vi "is-serial-port-open.vi"(11 "VISA Refnum in":refnum<visa-resource-name>) -> (0 "port-status":bool)   [LabVIEW 2024]
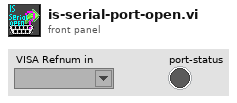
[diagram p1: front panel]
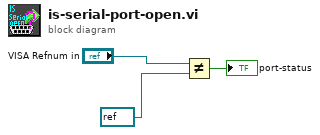
[diagram p0: block diagram]
diagram:
  n1 = Not Equal?(x="VISA Refnum in", y=refnum<visa-resource-name> refnum ("VISA resource name out")) -> (x != y?=→"port-status":bool)
